vi "ReadNetworkSettings.vi"(8 "error in (no error)":errorcluster, 11 "path":path) -> (0 "error out":errorcluster, 2 "found":bool, 3 "network settings":T1[](array[typedef]) {"IP Address Request Mode" items=["Static"=1, "DHCP/Link Local"=2, "Link-Local Only"=4, "DHCP Only"=8]; "Adapter Mode" items=["Disabled"=1, "TCP/IP Ethernet"=2, "Deterministic"=4, "EtherCAT"=8, "TCP/IP WLAN Connect"=32, "TCP/IP WLAN Create"=64]})   [LabVIEW 2017, in "USBDrive.lvlib"]
uses:
  <vilib>/addons/InsightCM/Devices/Shared/Common/USBDrive/USBDrive.lvlib
  <vilib>/addons/SystemInfoProcess/controls/NetworkAdapterSettings.ctl
  <vilib>/addons/SystemInfoProcess/SystemInfoProcess.lvlib
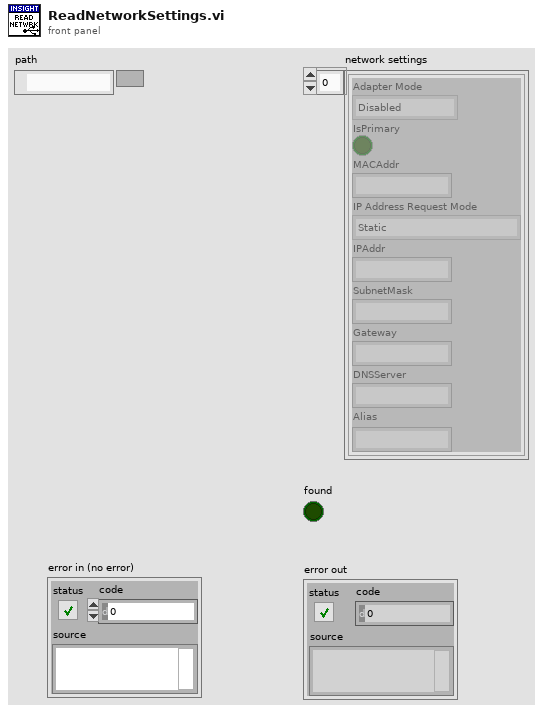
[diagram p1: front panel]
types:
  T1 = typedef "SystemInfoProcess.lvlib/NetworkAdapterSettings.ctl" = cluster{"Adapter Mode":u32, "IsPrimary":bool, "MACAddr":string, "IP Address Request Mode":u32, "IPAddr":string, "SubnetMask":string, "Gateway":string, "DNSServer":string, "Alias":string}
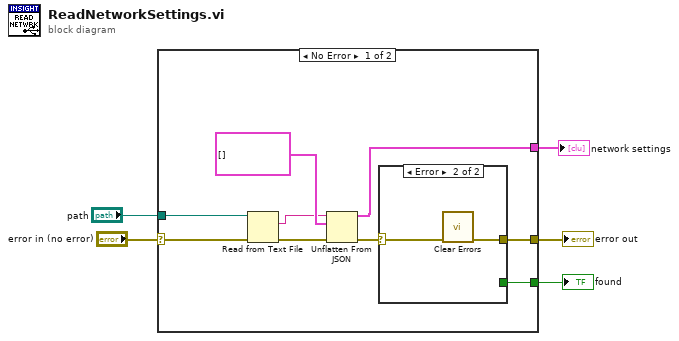
[diagram p0: block diagram]
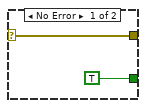
[diagram p2: hidden frame]
diagram:
  n1 = case shown="No Error" "error in (no error)" {
    selector: "error in (no error)" -> [w12 w19]
    tunnel: [w14 w19] -> w4
    tunnel: [w6 _] -> w1
    tunnel: [w13 _] -> w3
    tunnel: "path" -> [w11 _]
    frame No Error {
      n2 = Read from Text File(file (use dialog)=w11, error in=w12) -> (text=w7:string, error out=w10:errorcluster)  [unwired: 2 in, 2 out]
      n3 = Unflatten From JSON(JSON string=w7, type and defaults=T1[] [], error in (no error)=w10) -> (value=w6:T1[], error out=w9:errorcluster)  [unwired: 4 in]
      n4 = case shown="Error" w9 {
        selector: w9 -> [w16 w17]
        tunnel: [w16 w18] -> w14
        tunnel: [TRUE _] -> w13
        frame No Error {
        }
        frame Error {
          n5 = call <vilib>:"Clear Errors.vi"("error in (no error)"=w17) -> ("error out"=w18:errorcluster)  [unwired: 5 in, 1 out]
        }
      }
    }
    frame Error {
    }
  }
  "error out" <- w4
  "found" <- w3
  "network settings" <- w1
